vi "MELTPdll.vi"(8 "error in (no error)":errorcluster, 11 "Inputs":cluster{"p":dbl, "z":dbl[]}) -> (0 "error out":errorcluster, 3 "Outputs":T1)   [LabVIEW 2021]
doc: "subroutine MELTPdll(p, z, t, ierr, herr, herr_length)\n\nCompute the melting line temperature as a function of pressure and composition.\n\nINPUTS:\np -- Melting line pressure [kPa]\nz -- Composition (array of mole fractions)\n\nOUTPUTS:\nt -- Temperature [K] ierr, herr: See error codes in the ANCERR2 routine.\nierr -- error flag: 0 = successful\nherr -- error string\nherr_length -- length of variable herr (default: 255)"
uses:
  REFPROP.dll
panel:
  # "REFPROP-MELTPdll.vi"
  # "void  MELTPdll(double *p, double *z, double *t, int32_t *ierr, CStr herr, int32_t herr_length)"
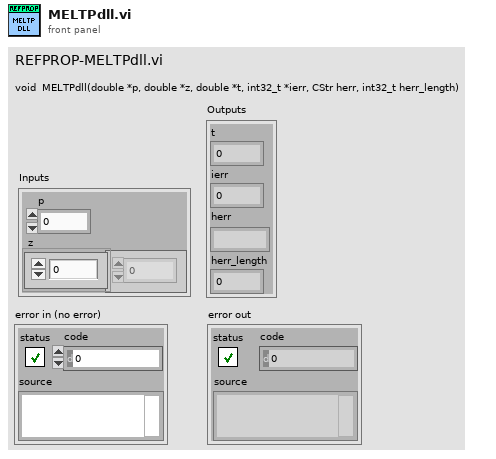
[diagram p1: front panel]
types:
  T1 = cluster{"t":dbl, "ierr":i32, "herr":string, "herr_length":i32}
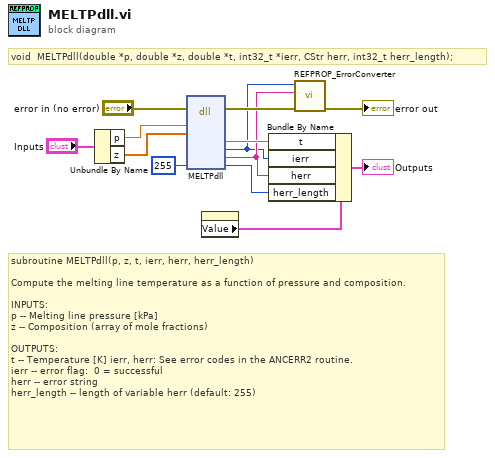
[diagram p0: block diagram]
diagram:
  # "void  MELTPdll(double *p, double *z, double *t, int32_t *ierr, CStr herr, int32_t herr_length);"
  # "subroutine MELTPdll(p, z, t, ierr, herr, herr_length)\n\nCompute the melting line temperature as a function of pressure and composition.\n\nINPUTS:\np -- Melting line pressure [kPa]\nz -- Composition (array of mole fractions)\n\nOUTPUTS:\nt -- Temperature [K] ierr, herr: See error codes in the ANCERR2 routine.\nierr -- error flag:  0 = successful\nherr -- error string\nherr_length -- length of variable herr (default: 255)"
  n1 = Unbundle By Name("Inputs") -> ("p"=w8:dbl, "z"=w7:dbl[])
  n2 = dll-call lib="C:/Users/lauria/OneDrive - National Institute of Standards and Technology (NIST)/LabVIEW Projects/7 REFPROP/REFPROP-wrappers-master/REFPROP-wrappers-master/wrappers/Labview/REFPROP/REFPROP.*" fn="MELTPdll"(error in="error in (no error)", "p"=w8, "z"=w7, "herr_length"=255 ("ln")) -> (error out=w12:errorcluster, "t"=w3:dbl, "ierr"=w1:i32, "herr"=w2:string, "herr_length"=w4:i32)  [unwired: 8 in, 1 out]
  n3 = property on="Outputs" class="Clust (strict)"() -> ("Value"=w5:T1)  [unwired: 2 in, 2 out]
  n4 = Bundle By Name(cluster=w5, "t"=w3, "ierr"=w1, "herr"=w2, "herr_length"=w4) -> (→"Outputs":T1)
  n5 = call "REFPROP_ErrorConverter.vi"("error in (no error)"=w12, "Error Message"=w2, "Error Code"=w1) -> ("error out"=→"error out":errorcluster)  [unwired: 8 in]
